vi "Teleop.vi"(10 "Match Info":T1={"Autonomous Elapsed Seconds"=0.0, "TeleOp Elapsed Seconds"=0.0, "Disabled Elapsed Seconds"=0.0, "Visited Autonomous"=FALSE, "Visited TeleOp"=FALSE, "Visited Disabled"=FALSE, "Autonomous Settings"={"Autonomous Style"=enum."Independent", "VI Refnum"=refnum}}, 11 "Call Context":T2) -> ()   [LabVIEW 2011]
doc: "This VI is called for each TeleOp packet received from the DS where the robot is not disabled. It is often used to read from the joysticks and update I/O or to update setpoints for timed control loops. It should complete and return within 20 milliseconds or it may miss DS packets."
uses:
  <vilib>/Rock Robotics/WPI/DriverStation/WPI_DriverStationDerivedRobotMode.ctl
  <vilib>/Rock Robotics/WPI/DriverStation/WPI_DriverStationMatch Info.ctl
  ControlModes.ctl
  Robot Global Data.vi
  <vilib>/Rock Robotics/WPI/Solenoid/Deprecated/WPI_SolenoidSetBool.vi
  <vilib>/Rock Robotics/WPI/Solenoid/Deprecated/WPI_SolenoidGetBool.vi
  AutoLevelStates.ctl
  VisionStates.ctl
  ShooterStates.ctl
panel:
  in  "Stage 2 Speed":dbl=1.0
  in  "Turret Speed":dbl=100.0
  in  "Backup Distance":dbl=6.0
  in  "Auto Level Backup Speed":dbl=-0.5
  in  "Auto Level Speed":dbl=0.5
  out "Waveform Chart 2":dbl(graph)
  out "Waveform Chart":dbl(graph)
  in  "Auto Level TD":u32=5
  out "Angular Rate":dbl
  out "Pitch":dbl
  in  "Auto Level Th (Deg/s)":dbl=5.0
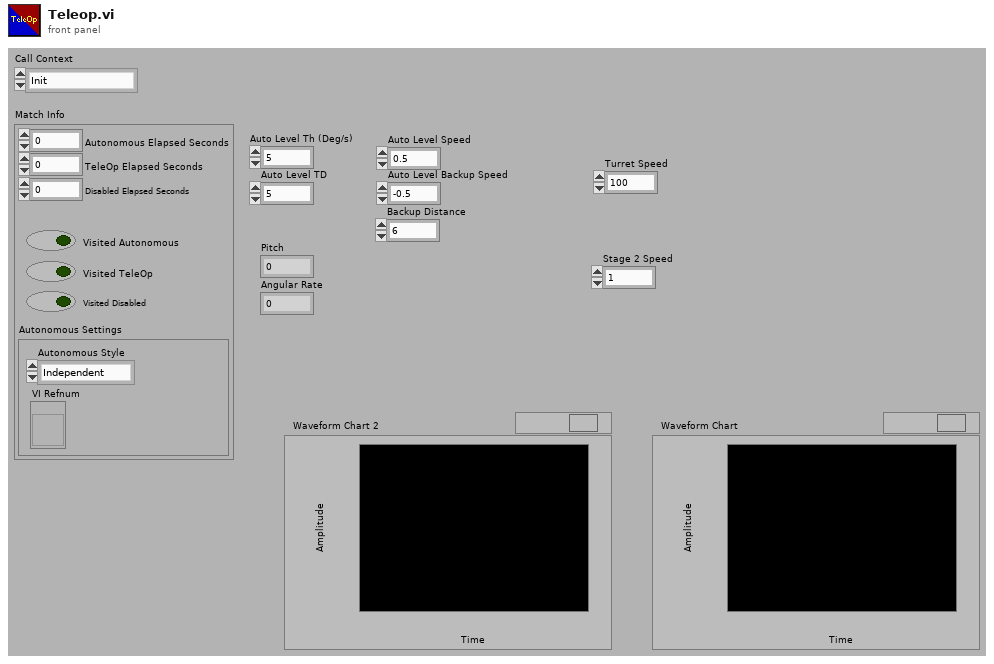
[diagram p1: front panel]
types:
  T1 = typedef "WPI_DriverStationMatch Info.ctl" = cluster{"Autonomous Elapsed Seconds":dbl, "TeleOp Elapsed Seconds":dbl, "Disabled Elapsed Seconds":dbl, "Visited Autonomous":bool, "Visited TeleOp":bool, "Visited Disabled":bool, "Autonomous Settings":cluster{"Autonomous Style":enum16{"Iterative", "Independent"}, "VI Refnum":refnum<vi>}}
  T2 = typedef "WPI_DriverStationDerivedRobotMode.ctl" = enum16{"Init", "Execute", "Stop"}
  T3 = typedef "ControlModes.ctl" = enum16{"Auto", "Key", "Fender", "Clearing"}
  T4 = typedef "AutoLevelStates.ctl" = enum16{"Manual", "AutoLevel", "Backup", "Hold"}
  T5 = typedef "WPI_GyroDevRef.ctl" = cluster{"DevStatus":errorcluster, "Analog Module":T6, "Analog Channel":T7, "Offset":dbl, "Gain (VoltsPerDegree/Second)":dbl}
  T6 = typedef "FPGA_TypedefAnalogModule.ctl" = enum16{"Analog Module 1", "Analog Module 2"}
  T7 = typedef "FPGA_AIChannel.ctl" = enum8{"AI 1", "AI 2", "AI 3", "AI 4", "AI 5", "AI 6", "AI 7", "AI 8", "Invalid"}
  T8 = typedef "Position Typedef.ctl" = cluster{"X":dbl, "Y":dbl, "Heading":dbl}
  T9 = typedef "WPI_RobotDriveDevRef.ctl" = cluster{"DevStatus":errorcluster, "Motors[]":T10[], "Square Inputs":bool, "Max Output":dbl, "Isochronous":bool}
  T10 = typedef "WPI_MotorControlDeviceRef.ctl" = cluster{"DeviceStatus":errorcluster, "Type":enum16{"PWM", "CAN"}, "PWM":cluster{"Digital Module":T11, "PWM Channel":T12, "DeadBand":T13}, "CAN":cluster{"Device Number":u8, "Control Mode":T14, "Semaphore":T15, "Max Vout":dbl}, "Invert":bool, "TransformRef":T16, "InvTransformRef":T16}
  T11 = typedef "FPGA_TypedefDigitalModule.ctl" = enum16{"Digital Module 1", "Digital Module 2"}
  T12 = typedef "FPGA_DIOPWMChannel.ctl" = enum8{"PWM 1", "PWM 2", "PWM 3", "PWM 4", "PWM 5", "PWM 6", "PWM 7", "PWM 8", "PWM 9", "PWM 10", "Invalid"}
  T13 = typedef "WPI_PWMDeadband.ctl" = cluster{"Name":string, "maxPositivePwm":i32, "minPositivePwm":i32, "centerPwm":i32, "maxNegativePwm":i32, "minNegativePwm":i32, "angularRange":u16}
  T14 = typedef "WPI_CANJaguar_ControlMode.ctl" = enum8{"Percent VBus", "Current", "Speed", "Position", "Voltage"}
  T15 = typedef "Semaphore RefNum" = refnum<k1>
  T16 = typedef "WPI_PWMTransform_ConPane.ctl" = refnum<vi>
  T17 = typedef "WPI_JoystickDevRef.ctl" = cluster{"Device":T18}
  T18 = typedef "WPI_JoystickDeviceEnum.ctl" = enum16{"USB 1", "USB 2", "USB 3", "USB 4", "Kinect 1", "Kinect 2"}
  T19 = typedef "WPI_JoystickButtonState.ctl" = cluster{"Button 1":bool, "Button 2":bool, "Button 3":bool, "Button 4":bool, "Button 5":bool, "Button 6":bool, "Button 7":bool, "Button 8":bool, "Button 9":bool, "Button 10":bool, "Button 11":bool, "Button 12":bool}
  T20 = cluster{"axis 1 (x)":dbl, "axis 2 (y)":dbl, "axis 3 (throttle)":dbl, "axis 4":dbl, "axis 5":dbl, "axis 6":dbl}
  T21 = typedef "VisionStates.ctl" = enum16{"Idle", "Aquiring", "Targeting", "Shooting"}
  T22 = typedef "ShooterStates.ctl" = enum16{"Wait", "Aquire", "SpinUp", "Shoot", "Test"}
  T23 = cluster{"Aquire Target":bool, "Target Aquired":bool, "Attempts":dbl}
  T24 = typedef "WPI_SolenoidDevRef.ctl" = cluster{"DevStatus":errorcluster, "Solenoid Module":T25, "Forward Solenoid Channel":T26, "Reverse Solenoid Channel":T26}
  T25 = typedef "FPGA_TypedefSolenoidModule.ctl" = enum16{"Solenoid Module 1", "Solenoid Module 2"}
  T26 = typedef "WPI_SolenoidChannel.ctl" = enum8{"Solenoid 1", "Solenoid 2", "Solenoid 3", "Solenoid 4", "Solenoid 5", "Solenoid 6", "Solenoid 7", "Solenoid 8", "Invalid"}
  T27 = typedef "CAN Data.ctl" = cluster{"Turret Position":dbl}
  T28 = typedef "WPI_EncoderDevRef.ctl" = cluster{"DevStatus":errorcluster, "EncoderIndex":T29, "CounterIndex":T30, "DistancePerCount":dbl, "Decoding Type":T31}
  T29 = typedef "FPGA_EncoderIdx.ctl" = enum8{"Enc 0", "Enc 1", "Enc 2", "Enc 3", "Invalid"}
  T30 = typedef "FPGA_CounterCtrSystemIndex.ctl" = enum8{"Ctr 0", "Ctr 1", "Ctr 2", "Ctr 3", "Ctr 4", "Ctr 5", "Ctr 6", "Ctr 7", "Invalid"}
  T31 = typedef "WPI_EncoderType.ctl" = enum16{"1x", "2x", "4x"}
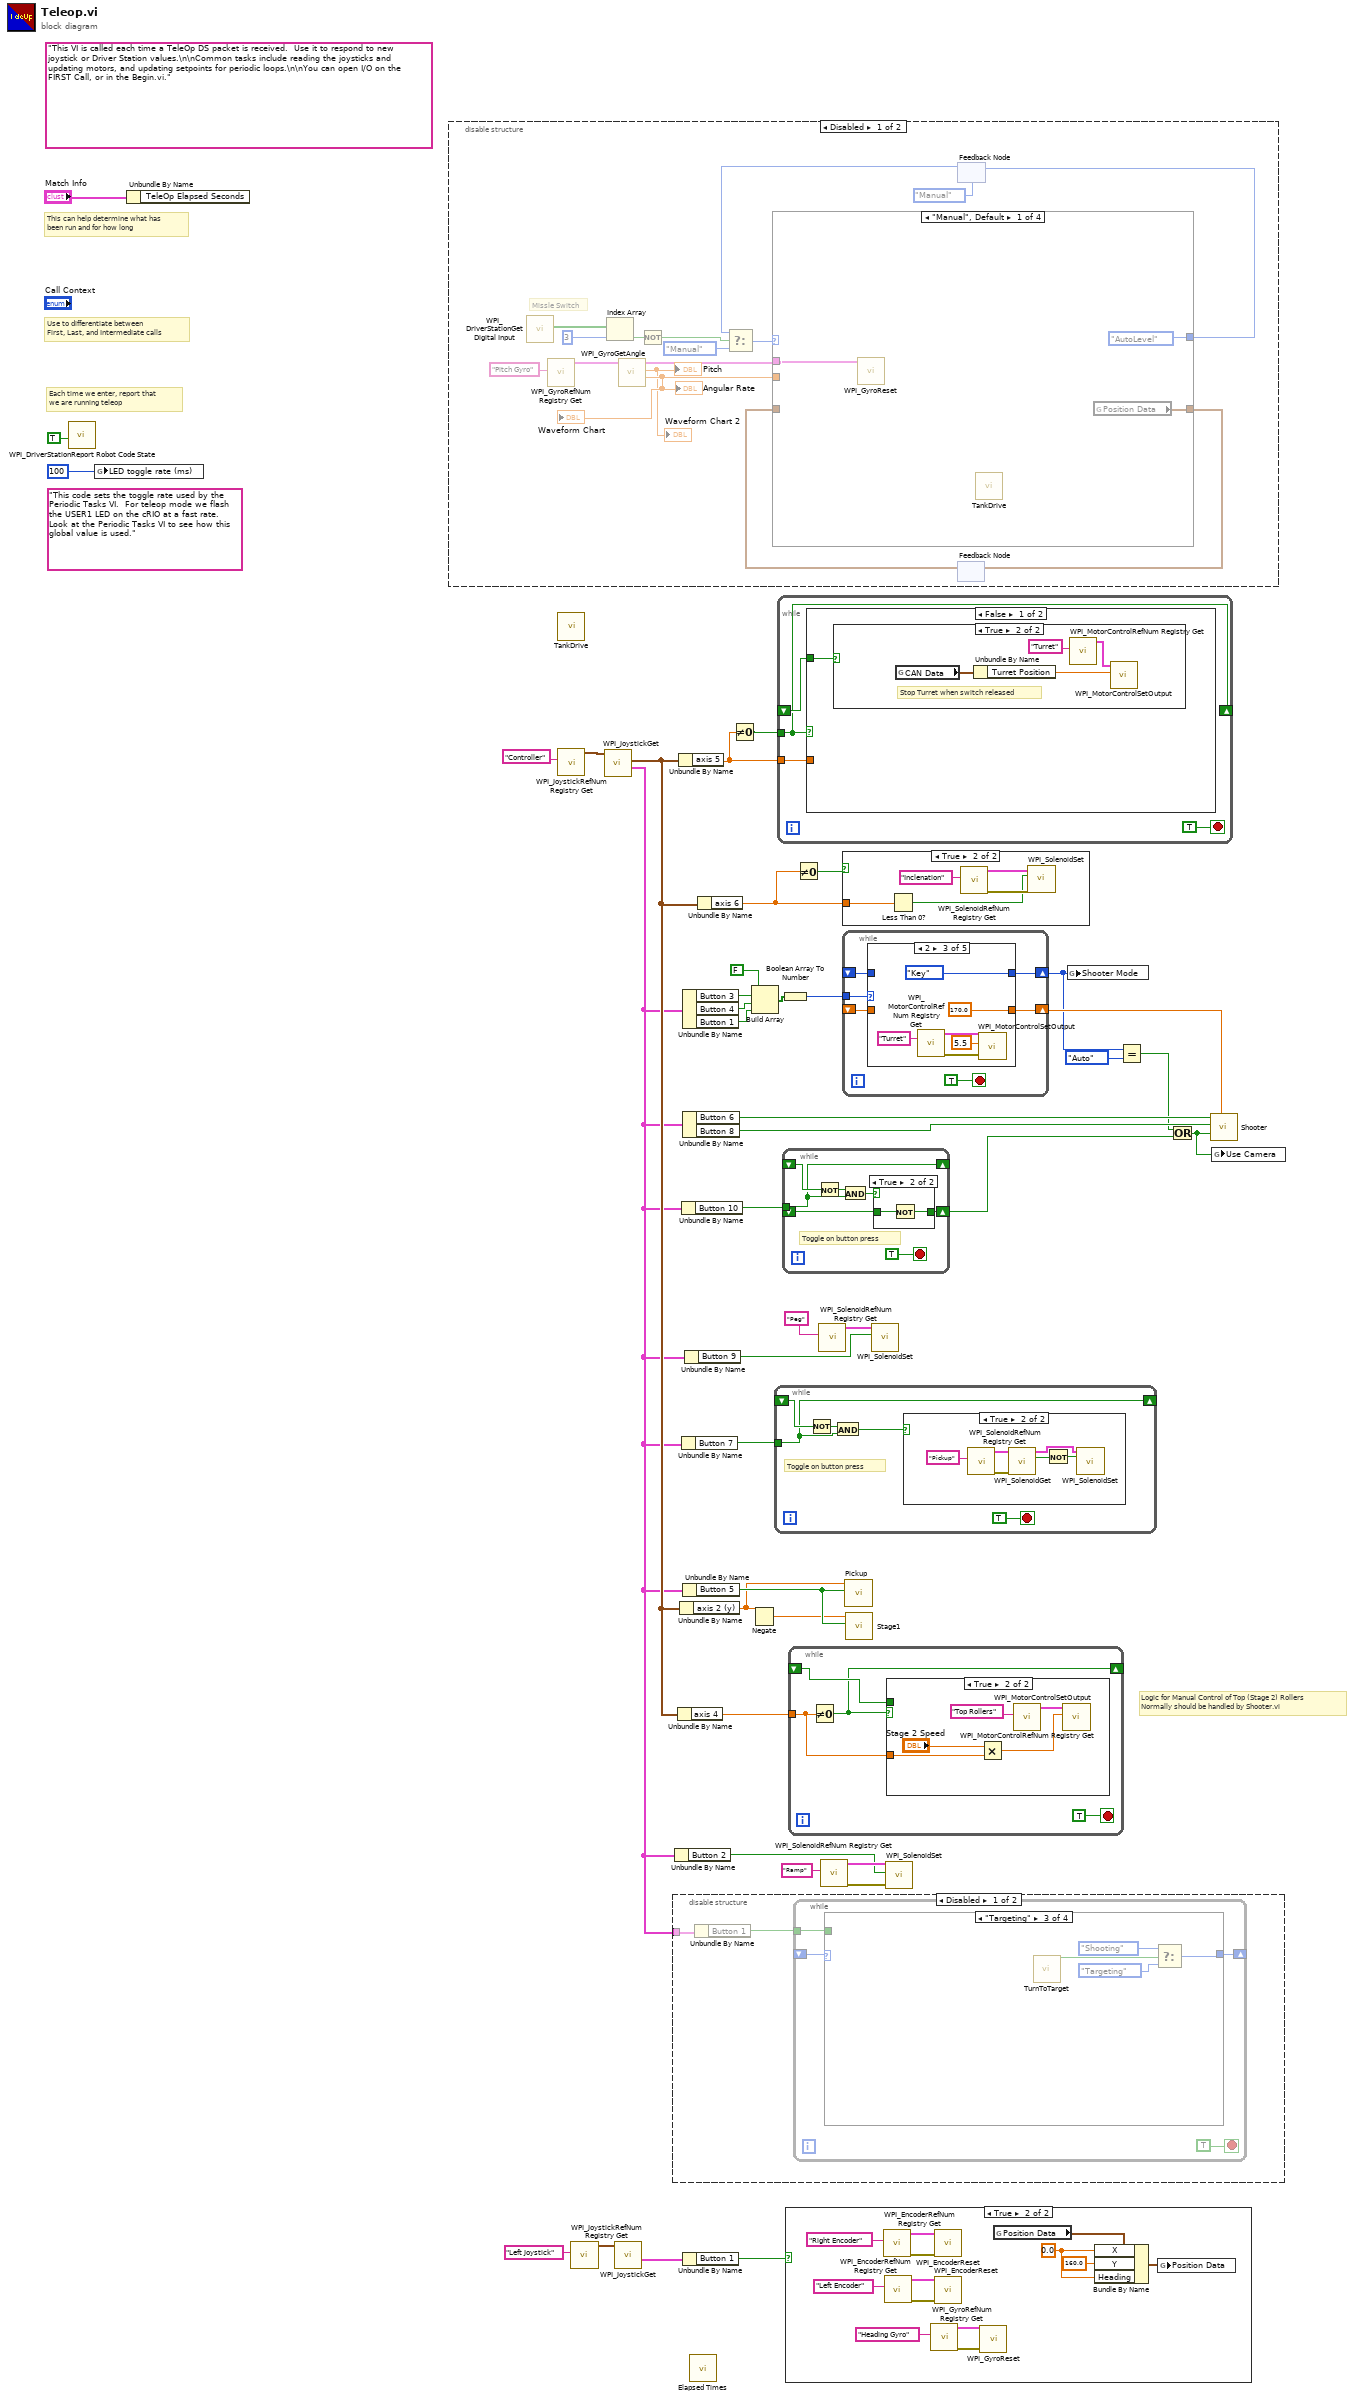
[diagram p0: block diagram]
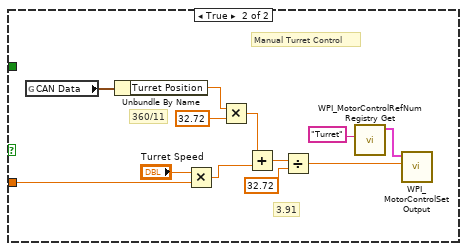
[diagram p4: hidden frame]
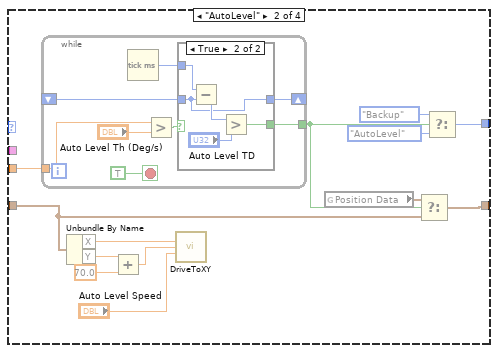
[diagram p5: hidden frame]
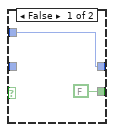
[diagram p6: hidden frame]
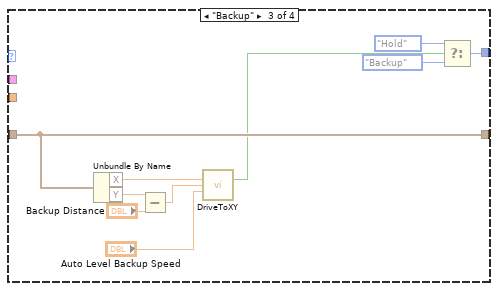
[diagram p7: hidden frame]
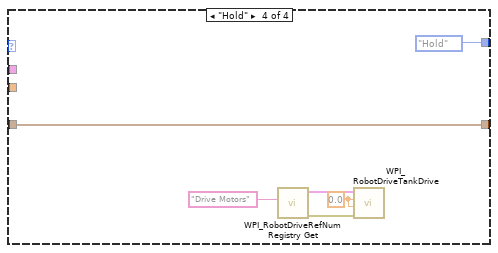
[diagram p8: hidden frame]
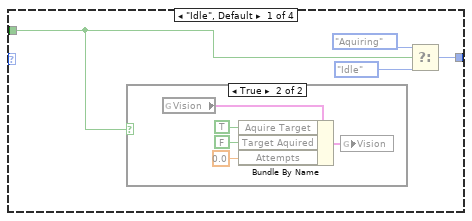
[diagram p11: hidden frame]
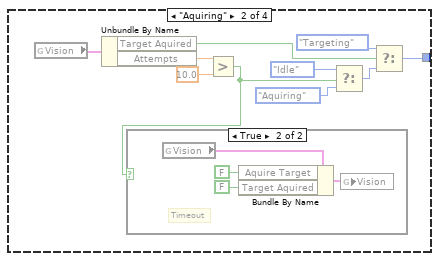
[diagram p13: hidden frame]
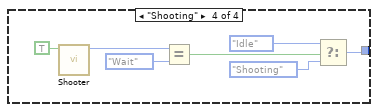
[diagram p15: hidden frame]
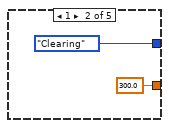
[diagram p18: hidden frame]
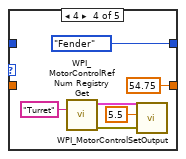
[diagram p19: hidden frame]
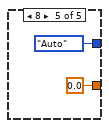
[diagram p20: hidden frame]
diagram:
  (unwired) "This code sets the toggle rate used by the Periodic Tasks VI.  For teleop mode we flash the USER1 LED on the cRIO at a fast rate.  Look at the Periodic Tasks VI to see how this global value is used."
  (unwired) "This VI is called each time a TeleOp DS packet is received.  Use it to respond to new joystick or Driver Station values.\n\nCommon tasks include reading the joysticks and updating motors, and updating setpoints for periodic loops.\n\nYou can open I/O on the FIRST Call, or in the Begin.vi."
  # "Logic for Manual Control of Top (Stage 2) Rollers\nNormally should be handled by Shooter.vi"
  # "Each time we enter, report that\nwe are running teleop"
  # "Use to differentiate between\nFirst, Last, and Intermediate calls"
  # "This can help determine what has\nbeen run and for how long"
  n1 = call <vilib>:"WPI_DriverStationReport Robot Code State.vi"("TeleOp"=TRUE ("Autonomous")) -> ()  [unwired: 10 in, 1 out]
  n2 = global write "Robot Global Data.vi" "LED toggle rate (ms)"(u32 100 ("LED ms toggle rate")) -> ()
  n3 = Unbundle By Name("Match Info") -> ()  [unwired: 1 out]
  n4 = disable-structure shown="Disabled" {
    frame Disabled {
      # "Missle Switch"
      n5 = call <vilib>:"WPI_DriverStationGet Digital Input.vi"() -> ("Driver Station Digital Input (1-8)"=w46:bool[])  [unwired: 11 out]
      n6 = call <vilib>:"WPI_GyroRefNum Registry Get.vi"("refnum name"="Pitch Gyro") -> ("GyroDevRef"=w52:T5)  [unwired: 9 in, 1 out]
      n7 = Index Array(array=w46, index=3) -> (element=w44:bool)
      n8 = call <vilib>:"WPI_GyroGetAngle.vi"("GyroDevRef"=w52) -> ("Angular Rate"=w48:dbl, "Angle"=→"Pitch" →"Waveform Chart 2":dbl, "GyroDevRef"=w51:T5)  [unwired: 7 in, 1 out]
      "Angular Rate" <- w48
      "Waveform Chart" <- w48
      n9 = Not(x=w44) -> (.not. x?=w43:bool)
      n10 = feedback #1() -> (w49:T8)  [unwired: 1 in]
      n11 = feedback #2(AutoLevelStates."Manual") -> (w54:T4)
      n12 = Select(t=w54, s=w43, f=AutoLevelStates."Manual") -> (s? t:f=w55:T4)
      n13 = case shown="\"Manual\", Default" w55 {
        tunnel: [AutoLevelStates."AutoLevel" w74 w97 AutoLevelStates."Hold"] -> w56
        tunnel: w51 -> [w61 _ _ _]
        tunnel: w48 -> [_ w71 _ _]
        tunnel: [w59 w65 w91 w100] -> w50
        tunnel: w49 -> [_ w64 w91 w100]
        frame "Manual", Default {
          n14 = call <vilib>:"WPI_GyroReset.vi"("GyroDevRef"=w61) -> ()  [unwired: 9 in, 2 out]
          n15 = call "TankDrive.vi"() -> ()  [unwired: 12 in]
          n16 = global read "Robot Global Data.vi" "Position Data"() -> (w59:T8)
        }
        frame "AutoLevel" {
          n17 = while {
            tunnel: w71 -> [w81]
            shift-right: [w79] -> _
            shift-left: _ -> [w77]
            tunnel: [w76] -> w62
            stop <- TRUE stop-if-true
            n18 = Tick Count (ms)() -> (millisecond timer value=w78:u32)
            n19 = Greater?(x=w81, y="Auto Level Th (Deg/s)") -> (0:w80:bool)
            n20 = case shown="True" w80 {
              tunnel: [w84 w86] -> w79
              tunnel: w78 -> [w84 w89]
              tunnel: w77 -> [_ w86]
              tunnel: [FALSE w85] -> w76
              frame False {
              }
              frame True {
                n21 = Subtract(x=w89, y=w86) -> (x-y=w88:u32)
                n22 = Greater?(x=w88, y="Auto Level TD") -> (0:w85:bool)
              }
            }
          }
          n23 = Unbundle By Name(w64) -> ("X"=w70:dbl, "Y"=w69:dbl)
          n24 = Add(x=w69, y=70.0) -> (x+y=w67:dbl)
          n25 = call "DriveToXY.vi"("X Target"=w70, "Y Target"=w67, "Speed"="Auto Level Speed") -> ()  [unwired: 10 in, 3 out]
          n26 = global read "Robot Global Data.vi" "Position Data"() -> (w63:T8)
          n27 = Select(t=w63, s=w62, f=w64) -> (s? t:f=w65:T8)
          n28 = Select(t=AutoLevelStates."Backup", s=w62, f=AutoLevelStates."AutoLevel") -> (s? t:f=w74:T4)
        }
        frame "Backup" {
          n29 = Unbundle By Name(w91) -> ("X"=w96:dbl, "Y"=w95:dbl)
          n30 = Subtract(x=w95, y="Backup Distance") -> (x-y=w93:dbl)
          n31 = call "DriveToXY.vi"("X Target"=w96, "Y Target"=w93, "Speed"="Auto Level Backup Speed") -> ("At Target"=w90:bool)  [unwired: 10 in, 2 out]
          n32 = Select(t=AutoLevelStates."Hold", s=w90, f=AutoLevelStates."Backup") -> (s? t:f=w97:T4)
        }
        frame "Hold" {
          w101 = 0.0 ("Left axis value")
          n33 = call <vilib>:"WPI_RobotDriveRefNum Registry Get.vi"("refnum name"="Drive Motors") -> ("error out"=w104:errorcluster, "RobotDriveDevRef"=w102:T9)  [unwired: 1 in, 8 out]
          n34 = call <vilib>:"WPI_RobotDriveTankDrive.vi"("error in (no error)"=w104, "Right axis value"=w101, "Left axis value"=w101, "RobotDriveDevRef"=w102) -> ()  [unwired: 6 in, 2 out]
        }
      }
      n35 = feedback-in #1(w50) -> ()
      n36 = feedback-in #2(w56) -> ()
    }
    frame Enabled {
    }
  }
  n37 = call "TankDrive.vi"() -> ()  [unwired: 12 in]
  n38 = call <vilib>:"WPI_JoystickRefNum Registry Get.vi"("refnum name"="Controller") -> ("JoystickDevRef"=w34:T17)  [unwired: 1 in, 9 out]
  n39 = call <vilib>:"WPI_JoystickRefNum Registry Get.vi"("refnum name"="Left Joystick") -> ("JoystickDevRef"=w38:T17)  [unwired: 1 in, 9 out]
  n40 = call <vilib>:"WPI_JoystickGet.vi"("JoystickDevRef"=w34) -> ("Buttons"=w7:T19, "Axes"=w25:T20)  [unwired: 1 in, 4 out]
  n41 = call <vilib>:"WPI_JoystickGet.vi"("JoystickDevRef"=w38) -> ("Buttons"=w37:T19)  [unwired: 1 in, 5 out]
  n42 = disable-structure shown="Disabled" {
    disable-tunnel: w7 -> [w106 _]
    frame Disabled {
      n43 = Unbundle By Name(w106) -> ("Button 1"=w107:bool)
      n44 = while {
        shift-right: [w110] -> _
        shift-left: _ -> [w109]
        tunnel: w107 -> [w108]
        stop <- TRUE stop-if-true
        n45 = case shown="\"Targeting\"" w109 {
          tunnel: [w113 w129 w138 w141] -> w110
          tunnel: w108 -> [w112 _ _ _]
          frame "Idle", Default {
            n46 = case shown="True" w112 {
              frame False {
              }
              frame True {
                n47 = global read "Robot Global Data.vi" "Vision"() -> (w119:T23)
                n48 = Bundle By Name(cluster=w119, "Aquire Target"=TRUE, "Target Aquired"=FALSE, "Attempts"=0.0) -> (w120:T23)
                n49 = global write "Robot Global Data.vi" "Vision"(w120) -> ()
              }
            }
            n50 = Select(t=VisionStates."Aquiring" ("Enum"), s=w112, f=VisionStates."Idle" ("Enum")) -> (s? t:f=w113:T21)
          }
          frame "Aquiring" {
            n51 = global read "Robot Global Data.vi" "Vision"() -> (w128:T23)
            n52 = Unbundle By Name(w128) -> ("Target Aquired"=w124:bool, "Attempts"=w127:dbl)
            n53 = Greater?(x=w127, y=10.0) -> (0:w122:bool)
            n54 = case shown="True" w122 {
              frame False {
              }
              frame True {
                # "Timeout"
                n55 = global read "Robot Global Data.vi" "Vision"() -> (w133:T23)
                n56 = Bundle By Name(cluster=w133, "Aquire Target"=FALSE, "Target Aquired"=FALSE) -> (w134:T23)
                n57 = global write "Robot Global Data.vi" "Vision"(w134) -> ()
              }
            }
            n58 = Select(t=VisionStates."Idle" ("Enum"), s=w122, f=VisionStates."Aquiring" ("Enum")) -> (s? t:f=w125:T21)
            n59 = Select(t=VisionStates."Targeting" ("Enum"), s=w124, f=w125) -> (s? t:f=w129:T21)
          }
          frame "Targeting" {
            n60 = call "TurnToTarget.vi"() -> ("On Target"=w136:bool)  [unwired: 11 in]
            n61 = Select(t=VisionStates."Shooting" ("Enum"), s=w136, f=VisionStates."Targeting" ("Enum")) -> (s? t:f=w138:T21)
          }
          frame "Shooting" {
            n62 = call "Shooter.vi"("Fire"=TRUE) -> ("Shooter State"=w145:T22)  [unwired: 9 in, 1 out]
            n63 = Equal?(x=w145, y=ShooterStates."Wait") -> (x = y?=w140:bool)
            n64 = Select(t=VisionStates."Idle" ("Enum"), s=w140, f=VisionStates."Shooting" ("Enum")) -> (s? t:f=w141:T21)
          }
        }
      }
    }
    frame Enabled {
    }
  }
  n65 = Unbundle By Name(w7) -> ("Button 2"=w29:bool)
  n66 = Unbundle By Name(w25) -> ("axis 4"=w28:dbl)
  n67 = Unbundle By Name(w25) -> ("axis 5"=w26:dbl)
  n68 = Unbundle By Name(w25) -> ("axis 2 (y)"=w9:dbl)
  n69 = Unbundle By Name(w7) -> ("Button 10"=w16:bool)
  n70 = Unbundle By Name(w7) -> ("Button 7"=w33:bool)
  n71 = Unbundle By Name(w7) -> ("Button 3"=w23:bool, "Button 4"=w22:bool, "Button 1"=w15:bool)
  n72 = Unbundle By Name(w37) -> ("Button 1"=w36:bool)
  n73 = Unbundle By Name(w7) -> ("Button 6"=w19:bool, "Button 8"=w18:bool)
  n74 = Unbundle By Name(w7) -> ("Button 5"=w24:bool)
  n75 = Unbundle By Name(w7) -> ("Button 9"=w4:bool)
  n76 = call "Elapsed Times.vi"() -> ()  [unwired: 3 in, 1 out]
  n77 = Unbundle By Name(w25) -> ("axis 6"=w2:dbl)
  n78 = Not Equal To 0?(x=w26) -> (x != 0?=w27:bool)
  n79 = Negate(x=w9) -> (-x=w10:dbl)
  n80 = Build Array(FALSE ("element"), w23, w22, w15) -> (w21:bool[])
  n81 = while {
    tunnel: w33 -> [w147]
    shift-right: [w147] -> _
    shift-left: _ -> [w149]
    stop <- TRUE stop-if-true
    # "Toggle on button press"
    n82 = Not(x=w149) -> (.not. x?=w148:bool)
    n83 = And(x=w148, y=w147) -> (x .and. y?=w146:bool)
    n84 = case shown="True" w146 {
      frame False {
      }
      frame True {
        n85 = call <vilib>:"WPI_SolenoidRefNum Registry Get.vi"("refnum name"="Pickup") -> ("error out"=w155:errorcluster, "SolenoidDevRef"=w154:T24)  [unwired: 9 in]
        n86 = call-poly <vilib>:"WPI_SolenoidGet.vi"("error in (no error)"=w155, "SolenoidDevRef"=w154) -> ("Value"=w152:bool, "SolenoidDevRef"=w151:T24)  [unwired: 7 in, 1 out]
        n87 = Not(x=w152) -> (.not. x?=w153:bool)
        n88 = call-poly <vilib>:"WPI_SolenoidSet.vi"("Value"=w153, "SolenoidDevRef"=w151) -> ()  [unwired: 8 in, 2 out]
      }
    }
  }
  n89 = while {
    tunnel: w27 -> [w158]
    tunnel: w26 -> [w160]
    shift-right: [w158] -> _
    shift-left: _ -> [w159]
    stop <- TRUE stop-if-true
    n90 = case shown="False" w158 {
      tunnel: w160 -> [_ w177]
      tunnel: w159 -> [w161 _]
      frame False {
        n91 = case shown="True" w161 {
          frame False {
          }
          frame True {
            # "Stop Turret when switch released"
            n92 = global read "Robot Global Data.vi" "CAN Data"() -> (w165:T27)
            n93 = Unbundle By Name(w165) -> ("Turret Position"=w162:dbl)
            n94 = call <vilib>:"WPI_MotorControlRefNum Registry Get.vi"("refnum name"="Turret") -> ("MotorControlDevRef"=w164:T10)  [unwired: 9 in, 1 out]
            n95 = call <vilib>:"WPI_MotorControlSetOutput.vi"("Output"=w162, "MotorControlDevRef"=w164) -> ()  [unwired: 8 in, 2 out]
          }
        }
      }
      frame True {
        # "Manual Turret Control"
        # "360/11"
        # "3.91"
        n96 = global read "Robot Global Data.vi" "CAN Data"() -> (w174:T27)
        n97 = Unbundle By Name(w174) -> ("Turret Position"=w167:dbl)
        n98 = Multiply(x="Turret Speed", y=w177) -> (x*y=w175:dbl)
        n99 = Multiply(x=w167, y=32.72) -> (x*y=w166:dbl)
        n100 = Add(x=w166, y=w175) -> (x+y=w173:dbl)
        n101 = Divide(x=w173, y=32.72) -> (x/y=w169:dbl)
        n102 = call <vilib>:"WPI_MotorControlRefNum Registry Get.vi"("refnum name"="Turret") -> ("MotorControlDevRef"=w171:T10)  [unwired: 9 in, 1 out]
        n103 = call <vilib>:"WPI_MotorControlSetOutput.vi"("Output"=w169, "MotorControlDevRef"=w171) -> ()  [unwired: 8 in, 2 out]
      }
    }
  }
  n104 = Boolean Array To Number(Boolean array=w21) -> (number=w20:u32)
  n105 = while {
    tunnel: w16 -> [w181]
    shift-right: [w181] -> _
    shift-left: _ -> [w183]
    shift-right: [w179] -> w14
    shift-left: _ -> [w178]
    stop <- TRUE stop-if-true
    # "Toggle on button press"
    n106 = Not(x=w183) -> (.not. x?=w182:bool)
    n107 = And(x=w182, y=w181) -> (x .and. y?=w180:bool)
    n108 = case shown="True" w180 {
      tunnel: [w185 w187] -> w179
      tunnel: w178 -> [w185 w186]
      frame False {
      }
      frame True {
        n109 = Not(x=w186) -> (.not. x?=w187:bool)
      }
    }
  }
  n110 = case shown="True" w36 {
    frame False {
    }
    frame True {
      w191 = 0.0 ("X")
      n111 = call <vilib>:"WPI_EncoderRefNum Registry Get.vi"("refnum name"="Right Encoder") -> ("error out"=w198:errorcluster, "EncoderDevRef"=w197:T28)  [unwired: 1 in, 8 out]
      n112 = call <vilib>:"WPI_EncoderRefNum Registry Get.vi"("refnum name"="Left Encoder") -> ("error out"=w195:errorcluster, "EncoderDevRef"=w196:T28)  [unwired: 1 in, 8 out]
      n113 = call <vilib>:"WPI_GyroRefNum Registry Get.vi"("refnum name"="Heading Gyro") -> ("error out"=w189:errorcluster, "GyroDevRef"=w188:T5)  [unwired: 1 in, 8 out]
      n114 = call <vilib>:"WPI_EncoderReset.vi"("error in (no error)"=w198, "EncoderDevRef"=w197) -> ()  [unwired: 8 in, 2 out]
      n115 = call <vilib>:"WPI_EncoderReset.vi"("error in (no error)"=w195, "EncoderDevRef"=w196) -> ()  [unwired: 8 in, 2 out]
      n116 = call <vilib>:"WPI_GyroReset.vi"("error in (no error)"=w189, "GyroDevRef"=w188) -> ()  [unwired: 8 in, 2 out]
      n117 = global read "Robot Global Data.vi" "Position Data"() -> (w194:T8)
      n118 = Bundle By Name(cluster=w194, "X"=w191, "Y"=160.0, "Heading"=w191) -> (w193:T8)
      n119 = global write "Robot Global Data.vi" "Position Data"(w193) -> ()
    }
  }
  n120 = while {
    tunnel: w28 -> [w201]
    shift-right: [w202] -> _
    shift-left: _ -> [w203]
    stop <- TRUE stop-if-true
    n121 = Not Equal To 0?(x=w201) -> (x != 0?=w202:bool)
    n122 = case shown="True" w202 {
      tunnel: w203 -> [w205 _]
      tunnel: w201 -> [_ w210]
      frame False {
        n123 = case shown="True" w205 {
          frame False {
          }
          frame True {
            n124 = call <vilib>:"WPI_MotorControlRefNum Registry Get.vi"("refnum name"="Top Rollers") -> ("MotorControlDevRef"=w207:T10)  [unwired: 9 in, 1 out]
            n125 = call <vilib>:"WPI_MotorControlSetOutput.vi"("Output"=0.0, "MotorControlDevRef"=w207) -> ()  [unwired: 8 in, 2 out]
          }
        }
      }
      frame True {
        n126 = Multiply(x="Stage 2 Speed", y=w210) -> (x*y=w209:dbl)
        n127 = call <vilib>:"WPI_MotorControlRefNum Registry Get.vi"("refnum name"="Top Rollers") -> ("MotorControlDevRef"=w212:T10)  [unwired: 9 in, 1 out]
        n128 = call <vilib>:"WPI_MotorControlSetOutput.vi"("Output"=w209, "MotorControlDevRef"=w212) -> ()  [unwired: 8 in, 2 out]
      }
    }
  }
  n129 = Not Equal To 0?(x=w2) -> (x != 0?=w3:bool)
  n130 = call <vilib>:"WPI_SolenoidRefNum Registry Get.vi"("refnum name"="Peg") -> ("SolenoidDevRef"=w5:T24)  [unwired: 9 in, 1 out]
  n131 = call <vilib>:"WPI_SolenoidRefNum Registry Get.vi"("refnum name"="Ramp") -> ("error out"=w31:errorcluster, "SolenoidDevRef"=w30:T24)  [unwired: 9 in]
  n132 = case shown="True" w3 {
    tunnel: w2 -> [_ w218]
    frame False {
    }
    frame True {
      n133 = Less Than 0?(x=w218) -> (x < 0?=w214:bool)
      n134 = call <vilib>:"WPI_SolenoidRefNum Registry Get.vi"("refnum name"="Inclenation") -> ("error out"=w215:errorcluster, "SolenoidDevRef"=w216:T24)  [unwired: 9 in]
      n135 = call-poly <vilib>:"WPI_SolenoidSet.vi"("error in (no error)"=w215, "Value"=w214, "SolenoidDevRef"=w216) -> ()  [unwired: 7 in, 2 out]
    }
  }
  n136 = while {
    tunnel: w20 -> [w224]
    shift-right: [w222] -> w13
    shift-left: _ -> [w221]
    shift-right: [w220] -> w17
    shift-left: _ -> [w219]
    stop <- TRUE stop-if-true
    n137 = case shown="2" w224 {
      tunnel: [w226 ControlModes."Clearing" ("Enum") ControlModes."Key" ("Enum") ControlModes."Fender" ("Enum") ControlModes."Auto" ("Enum")] -> w222
      tunnel: w221 -> [w226 _ _ _ _]
      tunnel: [w225 300.0 ("Distance") 170.0 ("Distance") 54.75 ("Distance") 0.0 ("Distance")] -> w220
      tunnel: w219 -> [w225 _ _ _ _]
      frame 0, Default {
      }
      frame 1 {
      }
      frame 2 {
        n138 = call <vilib>:"WPI_MotorControlRefNum Registry Get.vi"("refnum name"="Turret") -> ("error out"=w232:errorcluster, "MotorControlDevRef"=w231:T10)  [unwired: 9 in]
        n139 = call <vilib>:"WPI_MotorControlSetOutput.vi"("error in (no error)"=w232, "Output"=5.5, "MotorControlDevRef"=w231) -> ()  [unwired: 7 in, 2 out]
      }
      frame 4 {
        n140 = call <vilib>:"WPI_MotorControlRefNum Registry Get.vi"("refnum name"="Turret") -> ("error out"=w238:errorcluster, "MotorControlDevRef"=w237:T10)  [unwired: 9 in]
        n141 = call <vilib>:"WPI_MotorControlSetOutput.vi"("error in (no error)"=w238, "Output"=5.5, "MotorControlDevRef"=w237) -> ()  [unwired: 7 in, 2 out]
      }
      frame 8 {
      }
    }
  }
  n142 = call "Pickup.vi"("On?"=w24, "Pickup Speed"=w9) -> ()  [unwired: 10 in]
  n143 = call "Stage1.vi"("On?"=w24, "Stage 1 Speed"=w10) -> ()  [unwired: 10 in]
  n144 = call-poly <vilib>:"WPI_SolenoidSet.vi"("Value"=w4, "SolenoidDevRef"=w5) -> ()  [unwired: 8 in, 2 out]
  n145 = call-poly <vilib>:"WPI_SolenoidSet.vi"("error in (no error)"=w31, "Value"=w29, "SolenoidDevRef"=w30) -> ()  [unwired: 7 in, 2 out]
  n146 = global write "Robot Global Data.vi" "Shooter Mode"(w13) -> ()
  n147 = Equal?(x=w13, y=ControlModes."Auto") -> (x = y?=w11:bool)
  n148 = Or(x=w11, y=w14) -> (x .or. y?=w1:bool)
  n149 = call "Shooter.vi"("Distance"=w17, "Use Camera"=w1, "Test"=w18, "Fire"=w19) -> ()  [unwired: 6 in, 2 out]
  n150 = global write "Robot Global Data.vi" "Use Camera"(w1) -> ()
